vi "image_operations.vi"() -> ()   [LabVIEW 2024]
uses:
  <vilib>/vision/NI_Vision_Development_Module.lvlib
panel:
  in  "Dst Path":path
  out "Result Image":T1(plugin-control)
  out "Src Path":path
  out "String":string
  out "Y Resolution":i32
  out "X Resolution":i32
  out "File Data Type":i32(ring)=3 items=["1 bit", "2 bits", "4 bits", "8 bits", "12 bits (unsigned)", "16 bits (unsigned)", "16 bits (signed)", "16 bits (RGB chunky)", "24 bits (RGB chunky)", "24 bits (RGB planar)", "32 bits (unsigned)", "32 bits (signed)", "32 bits (RGB chunky)", "32 bits (float)", "48 bits (Complex 2x24 int)", "64 bits (Complex 2x32 float)", "reserved", "24 bits (HSL)", "48 bits (RGB chunky)", "64 bits (RGB chunky)"]
  out "Image Type":T2 items=["Grayscale (U8)", "Grayscale (I16)", "Grayscale (SGL)", "Complex (CSG)", "RGB (U32)", "HSL (U32)", "RGB (U64)", "Grayscale (U16)"]
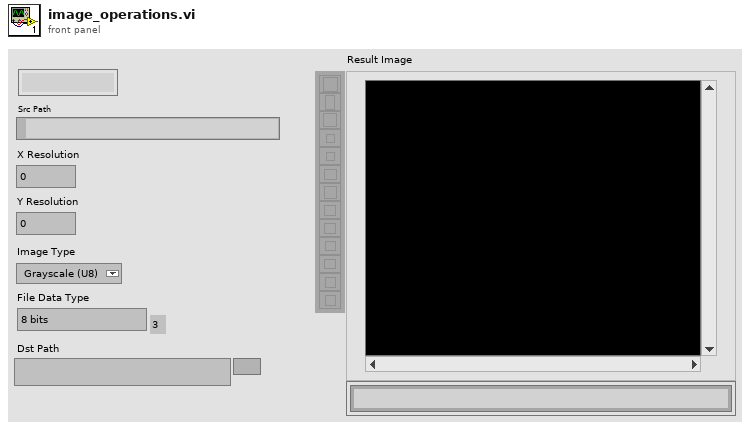
[diagram p1: front panel]
types:
  T1 = typedef "IMAQ Image.ctl" = refnum<image>
  T2 = typedef "Image Type" = u32
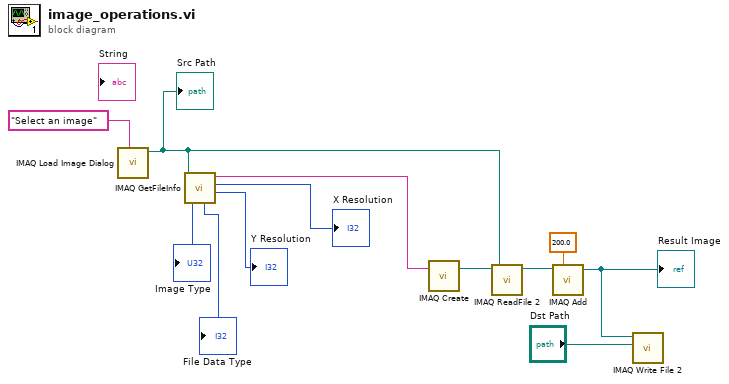
[diagram p0: block diagram]
diagram:
  n1 = call "IMAQ Load Image Dialog"("Prompt"="Select an image") -> ("Path"=w5:path)  [unwired: 8 in, 2 out]
  "Src Path" <- w5
  n2 = call "IMAQ GetFileInfo"("File Path"=w5) -> ("Y Resolution"=→"Y Resolution":i32, "X Resolution"=→"X Resolution":i32, "File Type"=w7:string, "File Data Type"=→"File Data Type":i32, "Image Type"=→"Image Type":T2)  [unwired: 4 in, 2 out]
  n3 = call "IMAQ Create"("Image Name"=w7) -> ("New Image"=w6:T1)  [unwired: 4 in, 1 out]
  n4 = call "IMAQ ReadFile 2"("File Path"=w5, "Image"=w6) -> ("Image Out"=w3:T1)  [unwired: 5 in, 4 out]
  n5 = call "IMAQ Add"("Image Src A"=w3, "Constant"=200.0) -> ("Image Dst Out"=w2:T1)  [unwired: 5 in, 1 out]
  "Result Image" <- w2
  n6 = call-poly "IMAQ Write File 2"("File Path"="Dst Path", "Image"=w2) -> ()  [unwired: 8 in, 2 out]
